vi "Init_queue.vi"(8 "error in (no error)":errorcluster, 9 "read queue":T1, 10 "Send queue":T2, 11 "QueueReader in":refnum<class "QueueReader.lvclass">) -> (0 "error out":errorcluster, 3 "QueueReader out":refnum<class "QueueReader.lvclass">)   [LabVIEW 2013, in "QueueReader.lvclass"]
doc: "Initializes the reader. Call before first use"
uses:
  QueueReader.lvclass
  message_queue.ctl
  Message/BaseMessage/BaseMessage.lvclass
  response queue.ctl
  response.ctl
  driver_status.ctl
  QueueReader.lvclass/QueueReader.ctl
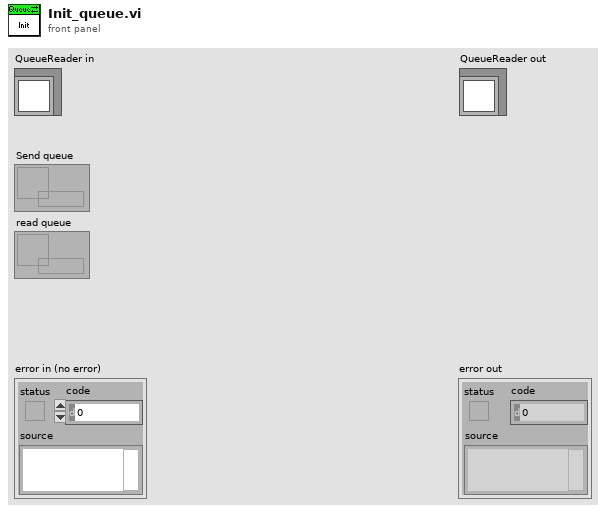
[diagram p1: front panel]
types:
  T1 = typedef "response queue.ctl" = refnum<queue>
  T2 = typedef "message_queue.ctl" = refnum<queue>
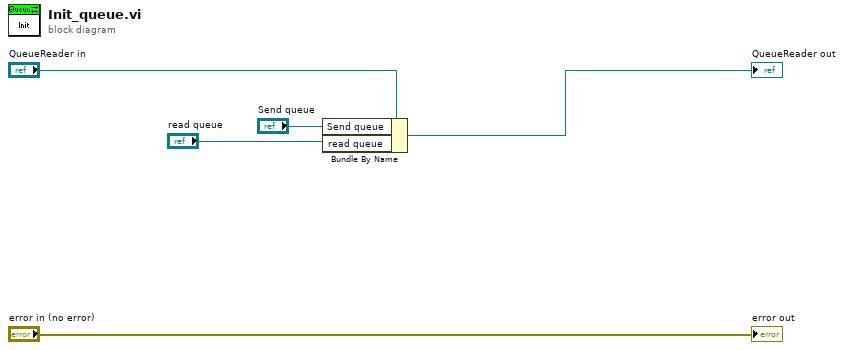
[diagram p0: block diagram]
diagram:
  n1 = Bundle By Name(cluster="QueueReader in", "Send queue"="Send queue", "read queue"="read queue") -> (→"QueueReader out":refnum<class "QueueReader.lvclass">)
  "error out" <- "error in (no error)"
